vi "20TVTI_Split_Cluster.vi"(0 "VTI Cluster":T1={"Temperatur (K)"=70.6986, "Setpoint (K)"=0.0, "Rate (K/min)"=3.4572, "Heater (%)"=0.0017142857142857142, "NV (%)"=0.0, "Heater Manual"=TRUE, "NV Manual"=TRUE, "Go to Set"=FALSE, "Pressure"=1.0208606, "Heater SP"=0.0, "Valid?"=FALSE, "Set Heater SP"=FALSE, "Set NV SP"=FALSE, "Heater (%) Display"=0.0, "NV (%) Display"=0.0, "NV Setpoint"=0.0, "Change Heater Status"=FALSE, "Change NV Status"=FALSE, "Change Sweep Type"=FALSE} {"NV (%) Display" format="%4_5f"; "Heater (%) Display" format="%4_5f"; "Heater SP" format="%#4_5f"; "Pressure" format="%#4_5f"; "NV (%)" scale=0.0..100.0; "Heater (%)" scale=0.0..100.0; "Rate (K/min)" format="%#4_5f"; "Setpoint (K)" format="%6_5f"}) -> (1 "VTI Status":T2={"Temperatur (K)"=70.6986, "Heater (%)"=0.0017142857142857142, "NV (%)"=0.0, "Heater Manual"=TRUE, "NV Manual"=TRUE, "Pressure"=1.0208606, "Dewar Pressure"=1.0500276, "Valid?"=FALSE, "Dewar Heater Manual"=FALSE, "Heater (%) Display"=0.0, "NV (%) Display"=0.0, "Dewar Heater (%)"=18.434412358753207, "D-Heater (%) Display"=18.434412358753207} {"Heater (%)" scale=0.0..100.0; "NV (%)" scale=0.0..100.0; "Dewar Heater (%)" scale=0.0..100.0}, 2 "VTI Control":T3)   [LabVIEW 2016]
uses:
  Gustav/20TVTI_Control.ctl
  Gustav/20TVTI_Status.ctl
  Gustav/20TVTI_Cluster.ctl
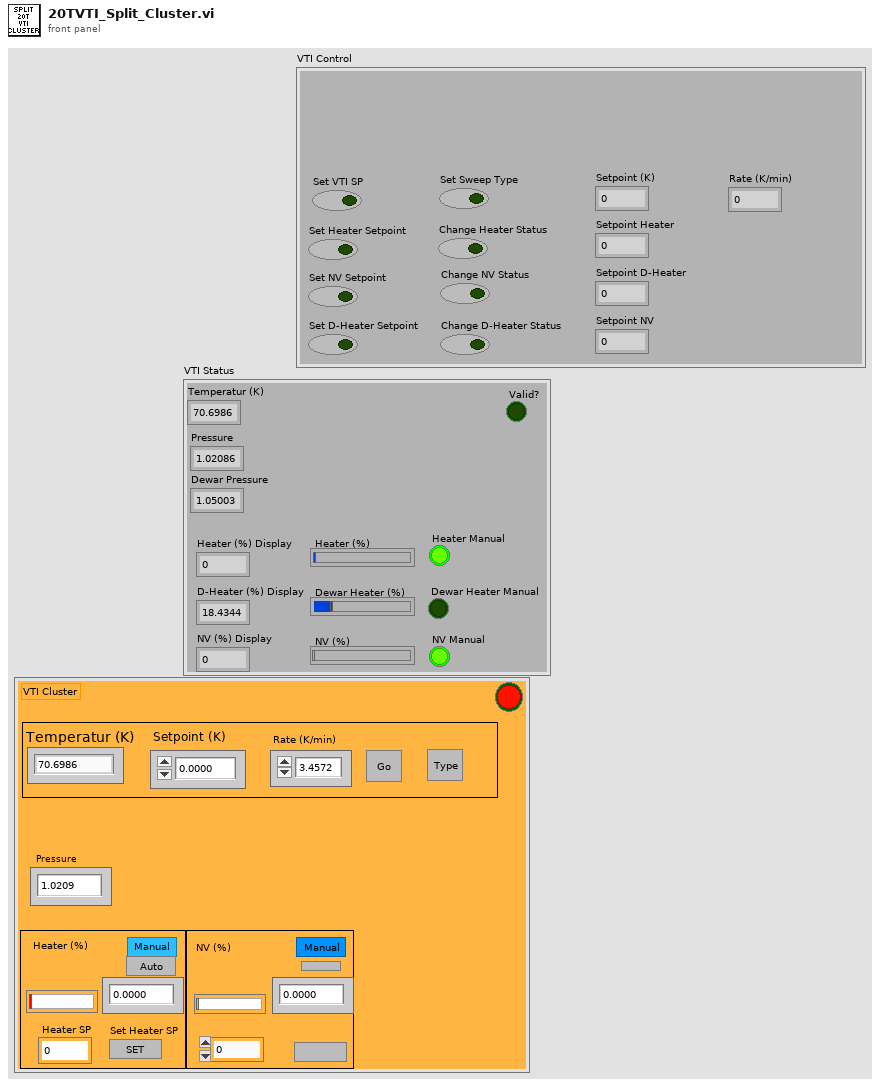
[diagram p1: front panel]
types:
  T1 = typedef "20TVTI_Cluster.ctl" = cluster{"Temperatur (K)":dbl, "Setpoint (K)":dbl, "Rate (K/min)":dbl, "Heater (%)":dbl, "NV (%)":dbl, "Heater Manual":bool, "NV Manual":bool, "Go to Set":bool, "Pressure":dbl, "Heater SP":dbl, "Valid?":bool, "Set Heater SP":bool, "Set NV SP":bool, "Heater (%) Display":dbl, "NV (%) Display":dbl, "NV Setpoint":dbl, "Change Heater Status":bool, "Change NV Status":bool, "Change Sweep Type":bool}
  T2 = typedef "20TVTI_Status.ctl" = cluster{"Temperatur (K)":dbl, "Heater (%)":dbl, "NV (%)":dbl, "Heater Manual":bool, "NV Manual":bool, "Pressure":dbl, "Dewar Pressure":dbl, "Valid?":bool, "Dewar Heater Manual":bool, "Heater (%) Display":dbl, "NV (%) Display":dbl, "Dewar Heater (%)":dbl, "D-Heater (%) Display":dbl}
  T3 = typedef "20TVTI_Control.ctl" = cluster{"Set VTI SP":bool, "Change NV Status":bool, "Set NV Setpoint":bool, "Change Heater Status":bool, "Set D-Heater Setpoint":bool, "Set Heater Setpoint":bool, "Change D-Heater Status":bool, "Set Sweep Type":bool, "Setpoint (K)":dbl, "Rate (K/min)":dbl, "Setpoint Heater":dbl, "Setpoint D-Heater":dbl, "Setpoint NV":dbl}
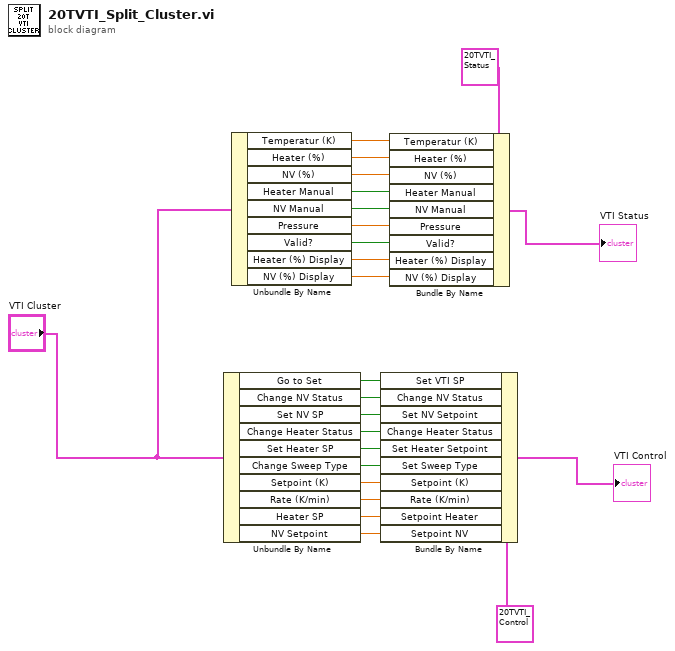
[diagram p0: block diagram]
diagram:
  n1 = Unbundle By Name("VTI Cluster") -> ("Go to Set"=w24:bool, "Change NV Status"=w23:bool, "Set NV SP"=w22:bool, "Change Heater Status"=w21:bool, "Set Heater SP"=w20:bool, "Change Sweep Type"=w19:bool, "Setpoint (K)"=w18:dbl, "Rate (K/min)"=w17:dbl, "Heater SP"=w16:dbl, "NV Setpoint"=w15:dbl)
  n2 = Unbundle By Name("VTI Cluster") -> ("Temperatur (K)"=w2:dbl, "Heater (%)"=w3:dbl, "NV (%)"=w4:dbl, "Heater Manual"=w5:bool, "NV Manual"=w6:bool, "Pressure"=w7:dbl, "Valid?"=w8:bool, "Heater (%) Display"=w9:dbl, "NV (%) Display"=w10:dbl)
  n3 = Bundle By Name(cluster=T3 {"Set VTI SP"=FALSE, "Change NV Status"=FALSE, "Set NV Setpoint"=FALSE, "Change Heater Status"=FALSE, "Set D-Heater Setpoint"=FALSE, "Set Heater Setpoint"=FALSE, "Change D-Heater Status"=FALSE, "Set Sweep Type"=FALSE, "Setpoint (K)"=0.0, "Rate (K/min)"=0.0, "Setpoint Heater"=0.0, "Setpoint D-Heater"=0.0, "Setpoint NV"=0.0} ("Cluster 3"), "Set VTI SP"=w24, "Change NV Status"=w23, "Set NV Setpoint"=w22, "Change Heater Status"=w21, "Set Heater Setpoint"=w20, "Set Sweep Type"=w19, "Setpoint (K)"=w18, "Rate (K/min)"=w17, "Setpoint Heater"=w16, "Setpoint NV"=w15) -> (→"VTI Control":T3)
  n4 = Bundle By Name(cluster=T2 {"Temperatur (K)"=70.6986, "Heater (%)"=0.0017142857142857142, "NV (%)"=0.0, "Heater Manual"=TRUE, "NV Manual"=TRUE, "Pressure"=1.0208606, "Dewar Pressure"=1.0500276, "Valid?"=FALSE, "Dewar Heater Manual"=FALSE, "Heater (%) Display"=0.0, "NV (%) Display"=0.0, "Dewar Heater (%)"=18.434412358753207, "D-Heater (%) Display"=18.434412358753207} ("VTI Status"), "Temperatur (K)"=w2, "Heater (%)"=w3, "NV (%)"=w4, "Heater Manual"=w5, "NV Manual"=w6, "Pressure"=w7, "Valid?"=w8, "Heater (%) Display"=w9, "NV (%) Display"=w10) -> (→"VTI Status":T2)
